vi "Lobatto Quadrature Core.vi"(8 "tolerance":dbl=1e-10, 9 "lower limit":dbl, 10 "upper limit":dbl, 11 "formula":string) -> (0 "error out":errorcluster, 3 "result":dbl)   [LabVIEW 2017, in "NI_AALPro.lvlib"]
uses:
  NI_AALPro.lvlib
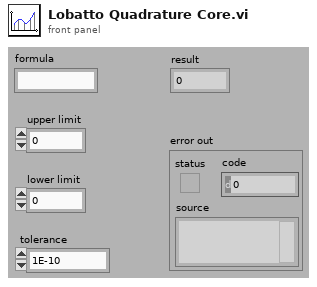
[diagram p1: front panel]
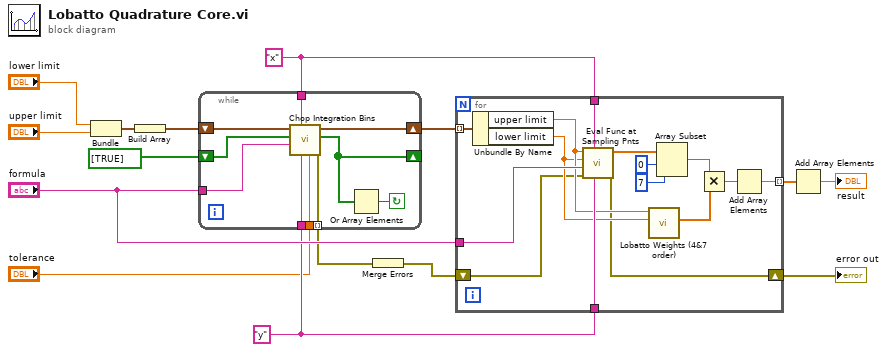
[diagram p0: block diagram]
diagram:
  w5 = "x" ("Variable Input")
  w7 = "y" ("Variable Output")
  n1 = Bundle("lower limit"="lower limit", "upper limit"="upper limit") -> (w13:cluster{"lower limit":dbl, "upper limit":dbl})  [unwired: 1 in]
  n2 = Build Array(w13) -> (w12:cluster{"lower limit":dbl, "upper limit":dbl}[])
  n3 = while {
    shift-right: [w24] -> w11
    shift-left: w12 -> [w25]
    shift-right: [w22] -> _
    shift-left: bool[] [TRUE] ("appended array") -> [w23]
    tunnel: w5 -> [w20]
    tunnel: "formula" -> [w19]
    tunnel: w7 -> [w18]
    tunnel: [w17] -> w2 mode=indexing
    tunnel: "tolerance" -> [w16]
    stop <- w21 continue-if-true
    n4 = call "Chop Integration Bins.vi"("tolerance"=w16, "variable output"=w18, "variable input"=w20, "formula"=w19, "Chop In"=w23, "Bins In"=w25) -> ("error out"=w17:errorcluster, "Chop Out"=w22:bool[], "Bins Out"=w24:cluster{"lower limit":dbl, "upper limit":dbl}[])  [unwired: 3 in]
    n5 = Or Array Elements(Boolean array=w22) -> (logical OR=w21:bool)
  }
  n6 = Merge Errors(w2) -> (w1:errorcluster)
  n7 = for {
    tunnel: w11 -> [w36] mode=indexing
    tunnel: w7 -> [w38]
    tunnel: "formula" -> [w37]
    tunnel: [w40] -> w10 mode=indexing
    tunnel: w5 -> [w39]
    shift-right: [w31] -> w3
    shift-left: w1 -> [w32]
    n8 = Unbundle By Name(w36) -> ("upper limit"=w35:dbl, "lower limit"=w34:dbl)
    n9 = call "Eval Func at Sampling Pnts.vi"("variable output"=w38, "variable input"=w39, "error in (no error)"=w32, "formula"=w37, "lower limit"=w34, "upper limit"=w35) -> ("error out"=w31:errorcluster, "Function Evaluations (7 and 4 pts)"=w30:dbl[])  [unwired: 3 in, 1 out]
    n10 = call "Lobatto Weights (4&7 order).vi"("lower limit"=w34, "upper limit"=w35) -> ("Weights (7-Order)"=w33:dbl[])  [unwired: 8 in, 1 out]
    n11 = Array Subset(array=w30, index=0, length=7) -> (w29:dbl[])
    n12 = Multiply(x=w29, y=w33) -> (x*y=w26:dbl[])
    n13 = Add Array Elements(numeric array=w26) -> (sum=w40:dbl)
  }
  "error out" <- w3
  n14 = Add Array Elements(numeric array=w10) -> (sum=→"result":dbl)
